vi "Save-Recall Instrument Settings.vi"(8 "error in (no error)":errorcluster, 9 "Memory Location (1)":u8=1, 10 "Operation (0: Save)":u16(ring) items=["Save", "Recall"], 11 "VISA resource name":refnum<visa-resource-name>) -> (0 "error out":errorcluster, 3 "VISA resource name out":refnum<visa-resource-name>)   [LabVIEW 2017, in "HH PLI Series.lvlib"]
doc: "Allows users to save or recall instrument setting."
uses:
  HH PLI Series.lvlib
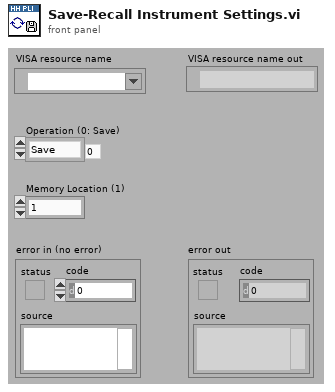
[diagram p1: front panel]
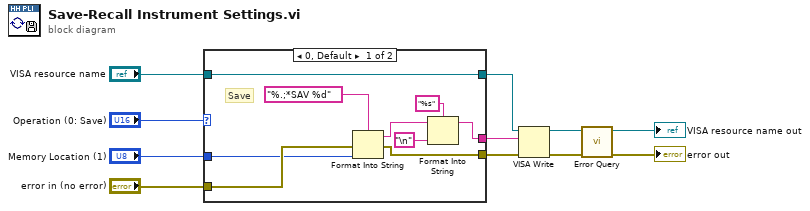
[diagram p0: block diagram]
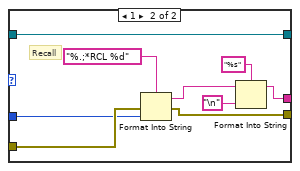
[diagram p2: hidden frame]
diagram:
  n1 = case shown="0, Default" "Operation (0: Save)" {
    tunnel: [w15 w23] -> w11
    tunnel: [w17 w28] -> w9
    tunnel: "error in (no error)" -> [w19 w29]
    tunnel: "Memory Location (1)" -> [w18 w26]
    tunnel: [w16 w25] -> w2
    tunnel: "VISA resource name" -> [w16 w25]
    frame 0, Default {
      # "Save"
      n2 = Format Into String(format string="%.;*SAV %d" ("command"), error in=w19, w18) -> (resulting string=w14:string, error out=w17:errorcluster)  [unwired: 1 in]
      n3 = Format Into String(format string="%s", initial string=w14, "\n") -> (resulting string=w15:string)  [unwired: 1 in, 1 out]
    }
    frame 1 {
      # "Recall"
      n4 = Format Into String(format string="%.;*RCL %d" ("command"), error in=w29, w26) -> (resulting string=w22:string, error out=w28:errorcluster)  [unwired: 1 in]
      n5 = Format Into String(format string="%s", initial string=w22, "\n") -> (resulting string=w23:string)  [unwired: 1 in, 1 out]
    }
  }
  n6 = VISA Write(VISA resource name=w2, write buffer=w11, error in (no error)=w9) -> (VISA resource name out=w6:refnum<visa-resource-name>, error out=w5:errorcluster)  [unwired: 1 out]
  n7 = call "Error Query.vi"("error in (no error)"=w5, "VISA resource name"=w6) -> ("error out"=→"error out":errorcluster, "VISA resource name out"=→"VISA resource name out":refnum<visa-resource-name>)  [unwired: 6 in, 2 out]
